vi "Define.vi"(11 "Definition":T1={"Type"={"Name"="", "Nullable"=FALSE, "Default NULL"=FALSE}, "Attributes"={"Primary Key"=FALSE, "Unique"=FALSE, "Foreign Key"=FALSE, "Auto Increment"=FALSE}, "String"={"Default"="", "Length"=255}}) -> (3 "String out":refnum<class "String.lvclass">)   [LabVIEW 2020, in "Conditu2.lvlib" / "Columns.lvlib" / "String.lvclass"]
uses:
  String.lvclass
  C:/dev/lv20CE/lv-conditum-tools/Conditum-Clone/Columns/Type/Type.lvclass
  String Definition.ctl
  Type/Definition.ctl
  Attributes.ctl
  Definition.ctl
  Field Type.ctl
  Type/Type.lvclass/Type.ctl
  String.lvclass/String.ctl
  Type/Type.lvclass
  Conditu2.lvlib
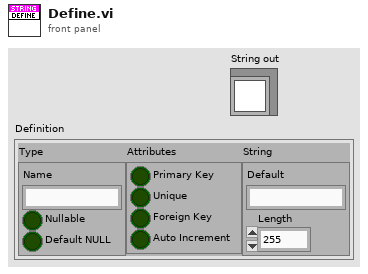
[diagram p1: front panel]
types:
  T1 = typedef "Conditu2.lvlib/Columns.lvlib/String.lvclass/String Definition.ctl" = cluster{"Type":T2, "Attributes":T3, "String":T4}
  T2 = typedef "Conditu2.lvlib/Columns.lvlib/Type.lvclass/Definition.ctl" = cluster{"Name":string, "Nullable":bool, "Default NULL":bool}
  T3 = typedef "Conditu2.lvlib/Attributes.ctl" = cluster{"Primary Key":bool, "Unique":bool, "Foreign Key":bool, "Auto Increment":bool}
  T4 = typedef "Conditu2.lvlib/Columns.lvlib/String.lvclass/Definition.ctl" = cluster{"Default":string, "Length":i32}
  T5 = typedef "Conditu2.lvlib/Field Type.ctl" = enum16{"None", "ID", "Boolean", "Integer", "Double", "Timestamp", "String", "Text", "Entity"}
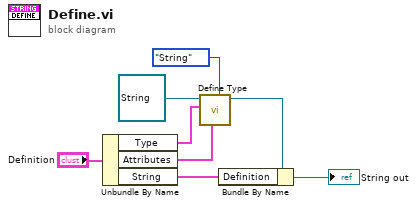
[diagram p0: block diagram]
diagram:
  n1 = Unbundle By Name("Definition") -> ("Type"=w6:T2, "Attributes"=w2:T3, "String"=w5:T4)
  n2 = call "Define Type.vi"("Type"=Field_Type."String", "Attributes"=w2, "Definition"=w6, "Type in"=refnum<class "String.lvclass"> refnum ("String out")) -> ("Type out"=w4:refnum<class "String.lvclass">)  [unwired: 7 in]
  n3 = Bundle By Name(cluster=w4, "Definition"=w5) -> (→"String out":refnum<class "String.lvclass">)
